vi "Recv().vi"(8 "Error In":errorcluster, 11 "Socket To Use":u32 format="%08x") -> (0 "Error Out":errorcluster, 1 "TimeStamp":u32, 2 "Bytes Read":i32, 3 "Socket Out":u32 format="%08x", 5 "Received IP Packet":u8[](array[numeric]) format="%02x")   [LabVIEW 2018]
uses:
  ws2_32.dll
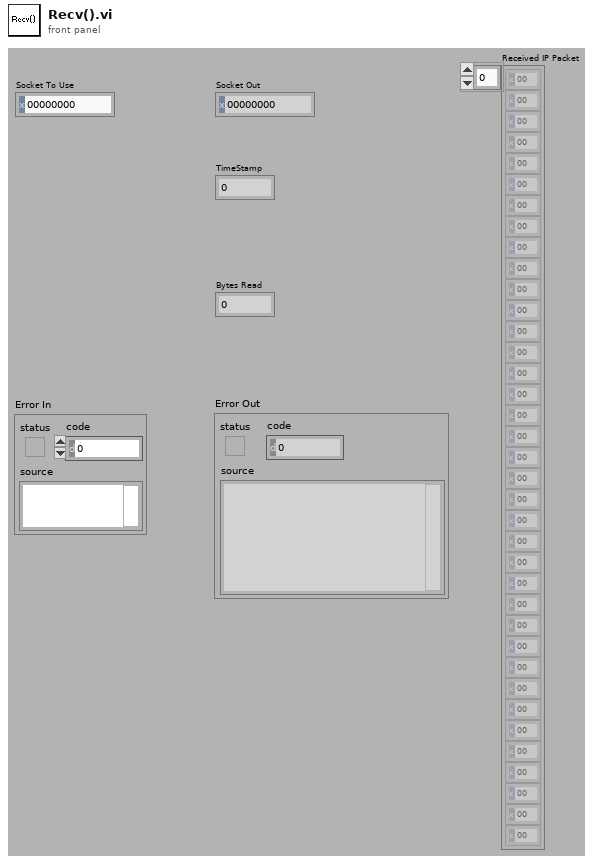
[diagram p1: front panel]
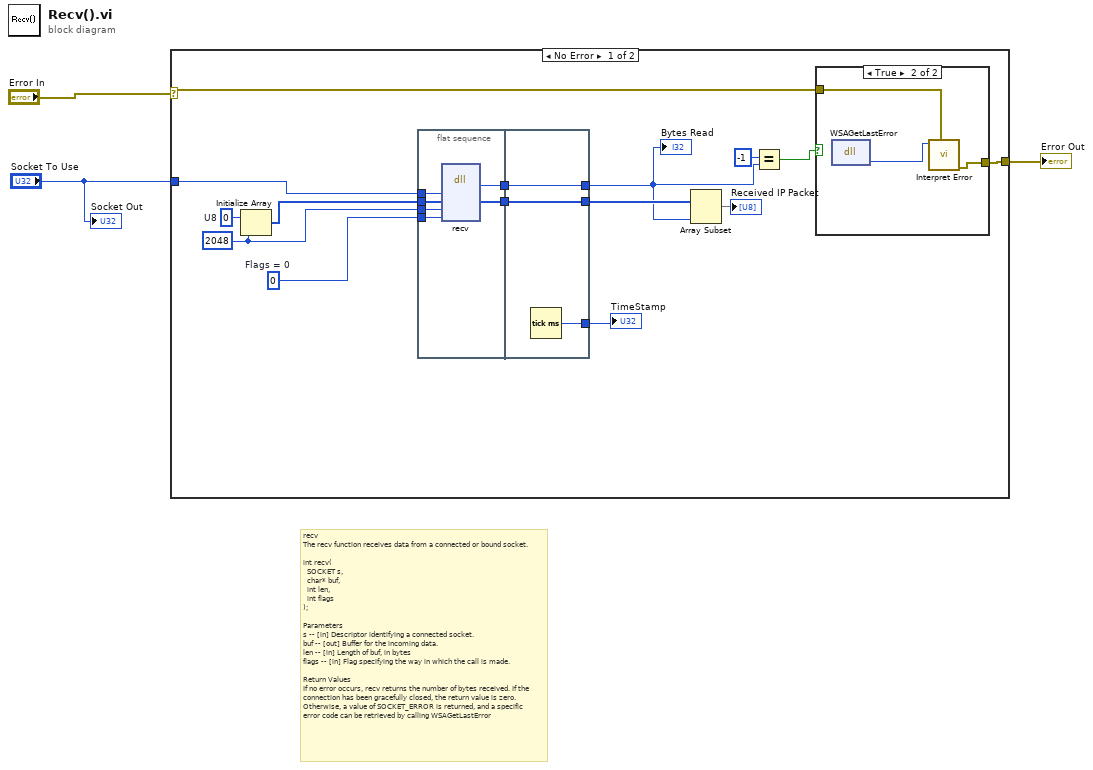
[diagram p0: block diagram]
diagram:
  # "recv\nThe recv function receives data from a connected or bound socket.\n\nint recv(\n  SOCKET s,\n  char* buf,\n  int len,\n  int flags\n);\n\nParameters\ns -- [in] Descriptor identifying a connected socket. \nbuf -- [out] Buffer for the incoming data. \nlen -- [in] Length of buf, in bytes \nflags -- [in] Flag specifying the way in which the call is made. \n\nReturn Values\nIf no error occurs, recv returns the number of bytes received. If the \nconnection has been gracefully closed, the return value is zero. \nOtherwise, a value of SOCKET_ERROR is returned, and a specific \nerror code can be retrieved by calling WSAGetLastError"
  n1 = case shown="No Error" "Error In" {
    selector: "Error In" -> [w8 w32]
    tunnel: [w12 w32] -> w3
    tunnel: "Socket To Use" -> [w4 _]
    frame No Error {
      w14 = u8 0  # U8
      w5 = 2048 ("dimension size")
      w15 = 0  # Flags = 0
      n2 = Initialize Array(w14, w5) -> (w13:u8[])
      n3 = flat-sequence {
        tunnel: w4 -> [w24]
        tunnel: w15 -> [w22]
        tunnel: w13 -> [w21]
        tunnel: w5 -> [w20]
        tunnel: [w23] -> w7
        tunnel: [w19] -> w6
        tunnel: [w25] -> w9
        tunnel: [w26] -> w10
        tunnel: [w27] -> w16
        tunnel: w7 -> [w27]
        tunnel: w6 -> [w26]
        frame #0 {
          n4 = dll-call lib="ws2_32.dll" fn="recv" label="recv()"("Socket to Use"=w24, "Receive Buffer"=w21, "Length of Buffer"=w20, "Flags"=w22) -> (w19:i32, "Receive Buffer"=w23:u8[])  [unwired: 6 in, 2 out]
        }
        frame #1 {
          n5 = Tick Count (ms)() -> (millisecond timer value=w25:u32)
        }
      }
      n6 = Array Subset(array=w16, length=w10) -> (→"Received IP Packet":u8[])  [unwired: 1 in]
      n7 = Equal?(x=-1, y=w10) -> (x = y?=w17:bool)
      n8 = case shown="True" w17 {
        tunnel: w8 -> [w28 w30]
        tunnel: [w28 w29] -> w12
        frame False {
        }
        frame True {
          n9 = dll-call lib="ws2_32.dll" fn="WSAGetLastError"() -> (w31:i32)  [unwired: 3 in, 2 out]
          n10 = call "Interpret Error.vi"("Error In"=w30, "Code"=w31) -> ("Error Out"=w29:errorcluster)  [unwired: 9 in]
        }
      }
      "Bytes Read" <- w10
      "TimeStamp" <- w9
    }
    frame Error {
    }
  }
  "Error Out" <- w3
  "Socket Out" <- "Socket To Use"
